vi "add new action to sequence.vi"(8 "error in (no error)":errorcluster, 9 "new action":refnum<class "action configuration.lvclass">, 10 "sequence name":string, 11 "Simple Sequencer TBM configuration in":refnum<class "Simple Sequencer TBM configuration.lvclass">) -> (0 "error out":errorcluster, 3 "Simple Sequencer TBM configuration out":refnum<class "Simple Sequencer TBM configuration.lvclass">)   [LabVIEW 2014, in "Simple Sequencer TBM configuration.lvclass"]
doc: "Adds the given action to the end of the specified sequence."
uses:
  Simple Sequencer TBM configuration.lvclass
  sequencer parent classes/action configuration parent/action configuration.lvclass
  Simple Sequencer TBM configuration.lvclass/Simple Sequencer TBM configuration.ctl
  <vilib>/NI/Configuration Framework/serializable configuration/NISE_CEF_serializable configuration.lvclass
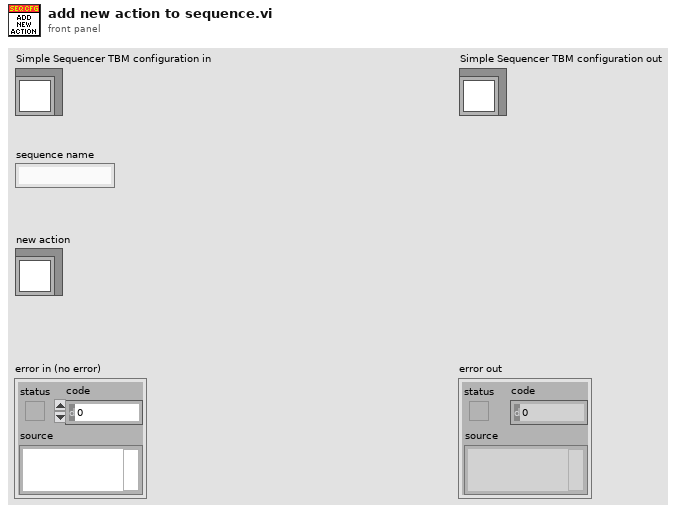
[diagram p1: front panel]
types:
  T1 = typedef "Simple Sequencer TBM configuration.lvclass/sequence definition.ctl" = cluster{"sequence name":string, "action configs":refnum<class "action configuration.lvclass">[]}
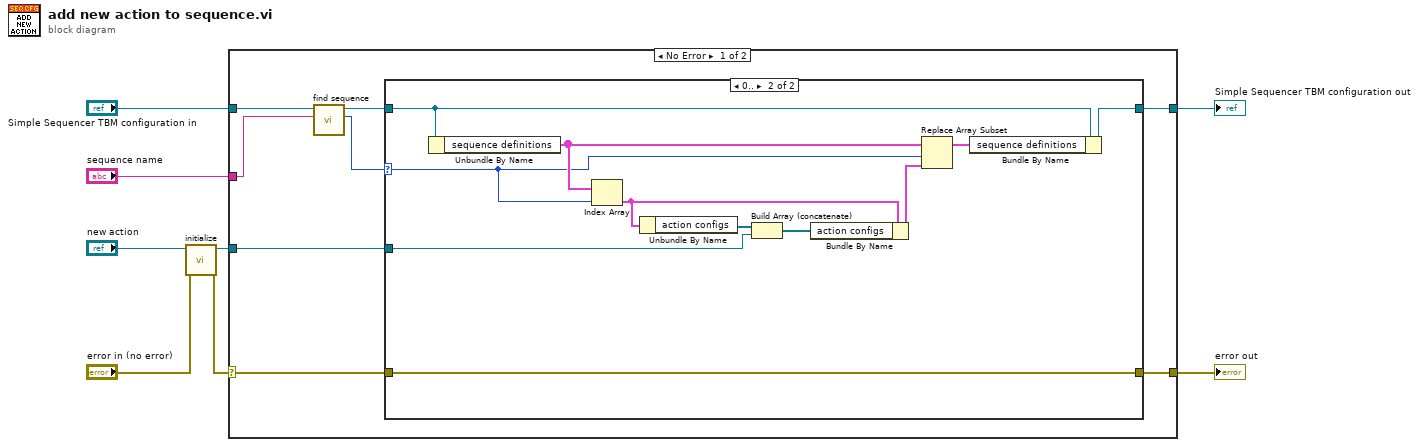
[diagram p0: block diagram]
diagram:
  n1 = call <vilib>:"initialize.vi"("error in"="error in (no error)", "configuration in"="new action") -> ("error out"=w2:errorcluster, "configuration out"=w1:refnum<class "action configuration.lvclass">)  [unwired: 7 in, 1 out]
  n2 = case shown="No Error" w2 {
    selector: w2 -> [w12 w31]
    tunnel: [w11 w31] -> w8
    tunnel: [w9 w30] -> w6
    tunnel: "Simple Sequencer TBM configuration in" -> [w16 w30]
    tunnel: "sequence name" -> [w15 _]
    tunnel: w1 -> [w10 _]
    frame No Error {
      n3 = call "find sequence.vi"("sequence name"=w15, "Simple Sequencer TBM configuration in"=w16) -> ("index"=w14:i32, "Simple Sequencer TBM configuration out"=w13:refnum<class "Simple Sequencer TBM configuration.lvclass">)  [unwired: 8 in]
      n4 = case shown="0.." w14 {
        selector: w14 -> [_ w23]
        tunnel: w13 -> [w17 w21]
        tunnel: w12 -> [w18 w29]
        tunnel: [w18 w29] -> w11
        tunnel: w10 -> [_ w27]
        tunnel: [w17 w19] -> w9
        frame ..-1 {
          # "#todo throw error not found"
        }
        frame 0.. {
          n5 = Unbundle By Name(w21) -> ("sequence definitions"=w24:T1[])
          n6 = Index Array(array=w24, index=w23) -> (element=w26:T1)
          n7 = Unbundle By Name(w26) -> ("action configs"=w28:refnum<class "action configuration.lvclass">[])
          n8 = Build Array (concatenate)(w28, w27) -> (w25:refnum<class "action configuration.lvclass">[])
          n9 = Bundle By Name(cluster=w26, "action configs"=w25) -> (w22:T1)
          n10 = Replace Array Subset(array=w24, new element=w22, index=w23) -> (w20:T1[])
          n11 = Bundle By Name(cluster=w21, "sequence definitions"=w20) -> (w19:refnum<class "Simple Sequencer TBM configuration.lvclass">)
        }
      }
    }
    frame Error {
    }
  }
  "error out" <- w8
  "Simple Sequencer TBM configuration out" <- w6
